vi "CLD 5 Parse Config Data File.vi"(8 "error in (no error)":errorcluster, 10 "Array In":T1[][](array[typedef])=[[{"Numeric"=1.25, "Boolean"=FALSE, "String"="One"}, {"Numeric"=1.35, "Boolean"=TRUE, "String"="Two"}, {"Numeric"=1.5, "Boolean"=FALSE, "String"="Three"}, {"Numeric"=1.0, "Boolean"=TRUE, "String"="Four"}], [{"Numeric"=2.0, "Boolean"=TRUE, "String"="Five"}, {"Numeric"=0.75, "Boolean"=FALSE, "String"="Six"}, {"Numeric"=0.9, "Boolean"=TRUE, "String"="Seven"}, {"Numeric"=0.75, "Boolean"=FALSE, "String"="Eight"}]], 11 "Get/Set":enum16{"Get", "Set"}(ring)) -> (0 "error out":errorcluster, 3 "Array Out":T1[][](array[typedef]))   [LabVIEW 2018]
doc: "CLD 5 exercise"
uses:
  CLD 5 Data Cluster.ctl
  <vilib>/Utility/config.llb/Read Key (Double).vi
  <vilib>/Utility/config.llb/Read Key (String).vi
  <vilib>/Utility/config.llb/Read Key (Boolean).vi
  <vilib>/Utility/config.llb/Read Key (I32).vi
  <vilib>/Utility/config.llb/Write Key (Double).vi
  <vilib>/Utility/config.llb/Write Key (Boolean).vi
  <vilib>/Utility/config.llb/Write Key (String).vi
  <vilib>/Utility/config.llb/Write Key (I32).vi
  <vilib>/Utility/config.llb/NI_LVConfig.lvlib
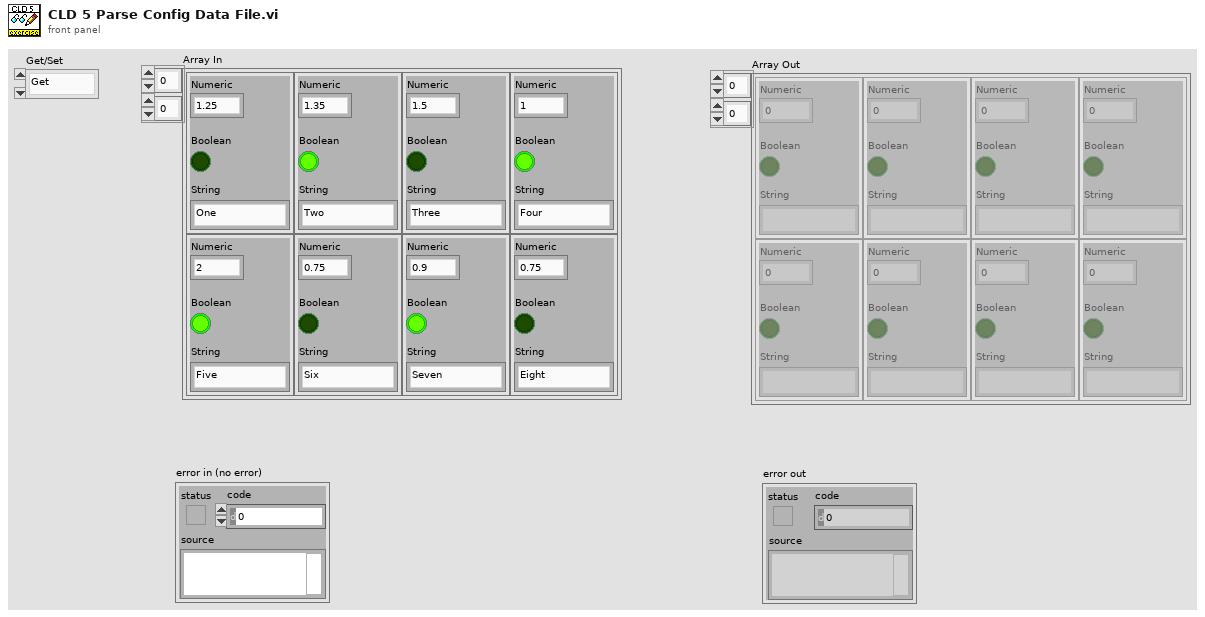
[diagram p1: front panel]
types:
  T1 = typedef "CLD 5 Data Cluster.ctl" = cluster{"Numeric":dbl, "Boolean":bool, "String":string}
  T2 = typedef "NI_LVConfig.lvlib/Config Data RefNum.ctl" = refnum<k1>
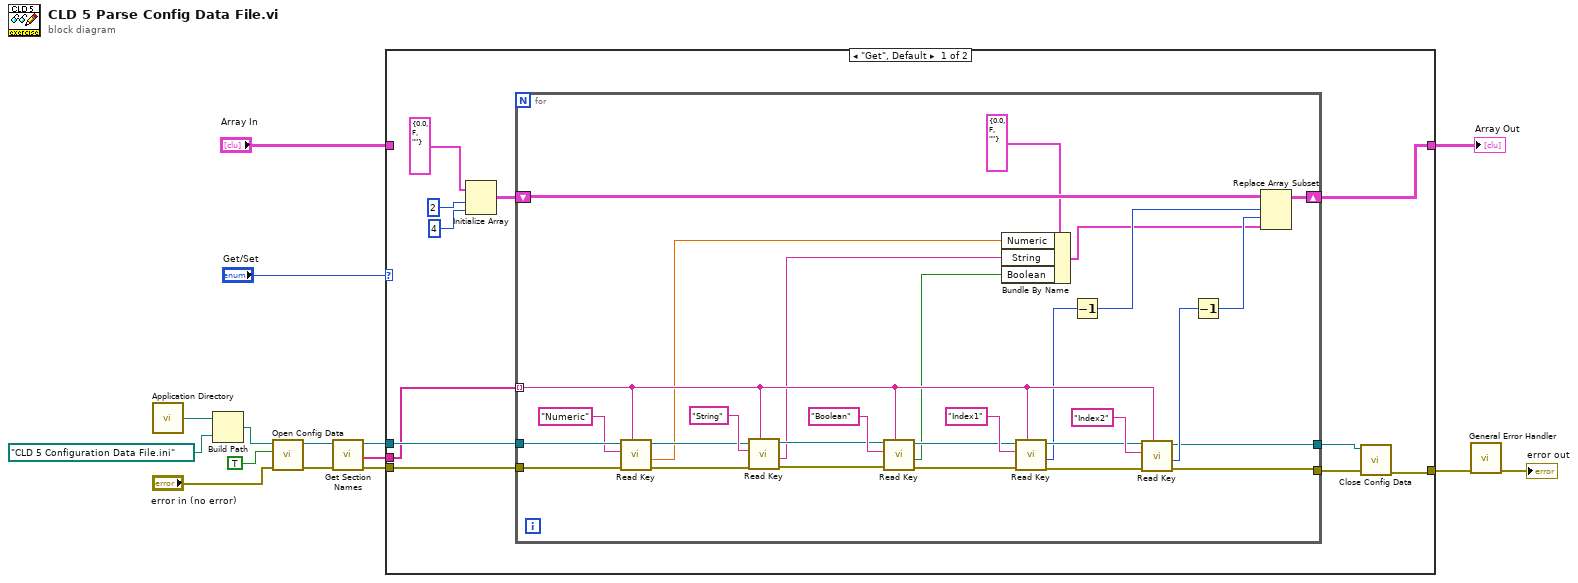
[diagram p0: block diagram]
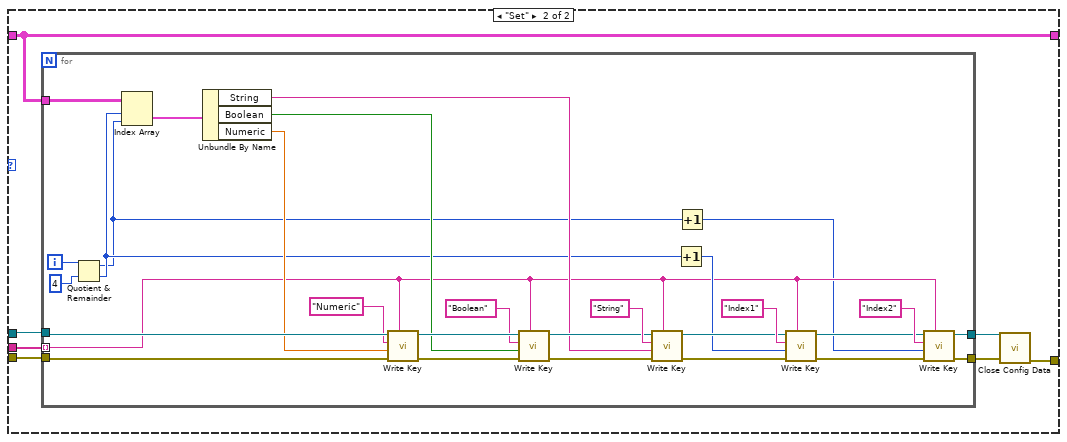
[diagram p2: hidden frame]
diagram:
  n1 = call <vilib>:"Application Directory.vi"() -> ("Application Directory"=w14:path)
  n2 = Build Path(base path=w14, name or relative path=path "CLD 5 Configuration Data File.ini") -> (appended path=w12:path)
  n3 = call <vilib>:"Open Config Data.vi"("error in (no error)"="error in (no error)", "create file if necessary (T)"=TRUE, "configuration file path"=w12) -> ("error out"=w10:errorcluster, "refnum"=w9:T2)  [unwired: 6 in, 1 out]
  n4 = call <vilib>:"Get Section Names.vi"("error in (no error)"=w10, "refnum"=w9) -> ("error out"=w6:errorcluster, "section names"=w7:string[], "refnum out"=w8:T2)  [unwired: 7 in]
  n5 = case shown="\"Get\", Default" "Get/Set" {
    tunnel: w8 -> [w26 w59]
    tunnel: w7 -> [w24 w62]
    tunnel: w6 -> [w25 w60]
    tunnel: [w17 w57] -> w2
    tunnel: [w19 w61] -> w4
    tunnel: "Array In" -> [_ w61]
    frame "Get", Default {
      n6 = Initialize Array(T1 {"Numeric"=0.0, "Boolean"=FALSE, "String"=""} ("Cluster"), 2 ("dimension size"), 4 ("dimension size")) -> (w21:T1[][])
      n7 = for {
        tunnel: w26 -> [w55]
        tunnel: w25 -> [w54]
        tunnel: w24 -> [w42] mode=indexing
        shift-right: [w38] -> w19
        shift-left: w21 -> [w39]
        tunnel: [w28] -> w18
        tunnel: [w27] -> w16
        n8 = call-poly <vilib>:"Read Key.vi"("section"=w42, "error in (no error)"=w54, "key"="Numeric", "refnum"=w55) -> ("error out"=w50:errorcluster, "value"=w32:dbl, "refnum out"=w51:T2)  [unwired: 4 in, 1 out]
        n9 = call-poly <vilib>:"Read Key.vi"("section"=w42, "error in (no error)"=w50, "key"="String", "refnum"=w51) -> ("error out"=w47:errorcluster, "value"=w31:string, "refnum out"=w48:T2)  [unwired: 4 in, 1 out]
        n10 = call-poly <vilib>:"Read Key.vi"("section"=w42, "error in (no error)"=w47, "key"="Boolean", "refnum"=w48) -> ("error out"=w44:errorcluster, "value"=w30:bool, "refnum out"=w45:T2)  [unwired: 4 in, 1 out]
        n11 = Bundle By Name(cluster=T1 {"Numeric"=0.0, "Boolean"=FALSE, "String"=""} ("Cluster"), "Numeric"=w32, "String"=w31, "Boolean"=w30) -> (w29:T1)
        n12 = call-poly <vilib>:"Read Key.vi"("section"=w42, "error in (no error)"=w44, "key"="Index1", "refnum"=w45) -> ("error out"=w40:errorcluster, "value"=w35:i32, "refnum out"=w41:T2)  [unwired: 4 in, 1 out]
        n13 = Decrement(x=w35) -> (x-1=w34:i32)
        n14 = call-poly <vilib>:"Read Key.vi"("section"=w42, "error in (no error)"=w40, "key"="Index2", "refnum"=w41) -> ("error out"=w28:errorcluster, "value"=w37:i32, "refnum out"=w27:T2)  [unwired: 4 in, 1 out]
        n15 = Decrement(x=w37) -> (x-1=w36:i32)
        n16 = Replace Array Subset(array=w39, new element=w29, index (row)=w34, index (col)=w36) -> (w38:T1[][])
      }
      n17 = call <vilib>:"Close Config Data.vi"("error in (no error)"=w18, "refnum"=w16) -> ("error out"=w17:errorcluster)  [unwired: 8 in, 1 out]
    }
    frame "Set" {
      n18 = for {
        tunnel: w62 -> [w67] mode=indexing
        tunnel: w61 -> [w91]
        tunnel: w60 -> [w86]
        tunnel: w59 -> [w87]
        tunnel: [w64] -> w58
        tunnel: [w63] -> w56
        i -> [w90]
        n19 = Quotient & Remainder(x=w90, y=4) -> (x-y*floor(x/y)=w66:i32, floor(x/y)=w72:i32)
        n20 = Index Array(array=w91, index (row)=w72, index (col)=w66) -> (element=w88:T1)
        n21 = Unbundle By Name(w88) -> ("String"=w76:string, "Boolean"=w80:bool, "Numeric"=w84:dbl)
        n22 = call-poly <vilib>:"Write Key.vi"("section"=w67, "error in (no error)"=w86, "value"=w84, "key"="Numeric", "refnum"=w87) -> ("error out"=w83:errorcluster, "refnum out"=w82:T2)  [unwired: 4 in, 1 out]
        n23 = call-poly <vilib>:"Write Key.vi"("section"=w67, "error in (no error)"=w83, "value"=w80, "key"="Boolean", "refnum"=w82) -> ("error out"=w78:errorcluster, "refnum out"=w77:T2)  [unwired: 4 in, 1 out]
        n24 = call-poly <vilib>:"Write Key.vi"("section"=w67, "error in (no error)"=w78, "value"=w76, "key"="String", "refnum"=w77) -> ("error out"=w74:errorcluster, "refnum out"=w73:T2)  [unwired: 4 in, 1 out]
        n25 = Increment(x=w72) -> (x+1=w71:i32)
        n26 = Increment(x=w66) -> (x+1=w65:i32)
        n27 = call-poly <vilib>:"Write Key.vi"("section"=w67, "error in (no error)"=w74, "value"=w71, "key"="Index1", "refnum"=w73) -> ("error out"=w68:errorcluster, "refnum out"=w69:T2)  [unwired: 4 in, 1 out]
        n28 = call-poly <vilib>:"Write Key.vi"("section"=w67, "error in (no error)"=w68, "value"=w65, "key"="Index2", "refnum"=w69) -> ("error out"=w64:errorcluster, "refnum out"=w63:T2)  [unwired: 4 in, 1 out]
      }
      n29 = call <vilib>:"Close Config Data.vi"("error in (no error)"=w58, "refnum"=w56) -> ("error out"=w57:errorcluster)  [unwired: 8 in, 1 out]
    }
  }
  "Array Out" <- w4
  n30 = call <vilib>:"General Error Handler.vi"("error in (no error)"=w2) -> ("error out"=→"error out":errorcluster)  [unwired: 10 in, 4 out]
